vi "Write Voffset.vi"(8 "error in (no error)":errorcluster, 10 "Voffset":dbl, 11 "Update Speaker Vscale CMD in":refnum<class "Update Speaker Vscale CMD.lvclass">) -> (0 "error out":errorcluster, 3 "Update Speaker Vscale CMD out":refnum<class "Update Speaker Vscale CMD.lvclass">)   [LabVIEW 2016, in "gPAS Library.lvlib" / "Update Speaker Vscale CMD.lvclass"]
uses:
  Update Speaker Vscale CMD.lvclass
  Update Speaker Vscale CMD.lvclass/Update Speaker Vscale CMD.ctl
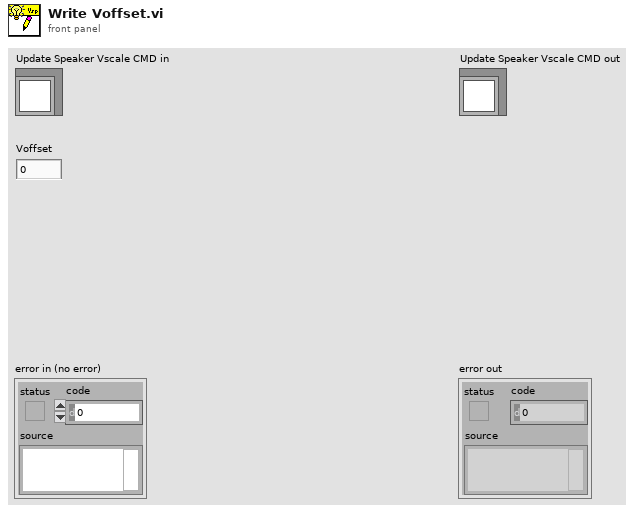
[diagram p1: front panel]
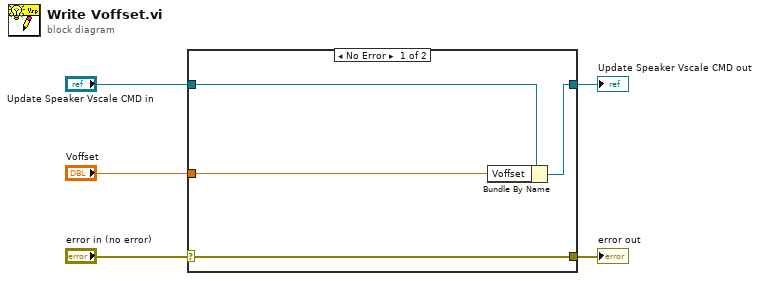
[diagram p0: block diagram]
diagram:
  n1 = case shown="No Error" "error in (no error)" {
    selector: "error in (no error)" -> [w9 w10]
    tunnel: [w9 w10] -> w4
    tunnel: [w7 w11] -> w2
    tunnel: "Update Speaker Vscale CMD in" -> [w8 w11]
    tunnel: "Voffset" -> [w6 _]
    frame No Error {
      n2 = Bundle By Name(cluster=w8, "Voffset"=w6) -> (w7:refnum<class "Update Speaker Vscale CMD.lvclass">)
    }
    frame Error {
    }
  }
  "error out" <- w4
  "Update Speaker Vscale CMD out" <- w2
